vi "Write Scanner UDP Handle.vi"(8 "error in (no error)":errorcluster, 10 "HTTP response":string, 11 "PF_API in":refnum<class "PF_API.lvclass">) -> (0 "error out":errorcluster, 3 "PF_API out":refnum<class "PF_API.lvclass">)   [LabVIEW 2019, in "PF_API.lvclass"]
uses:
  PF_API.lvclass
  PF_API.lvclass/PF_API.ctl
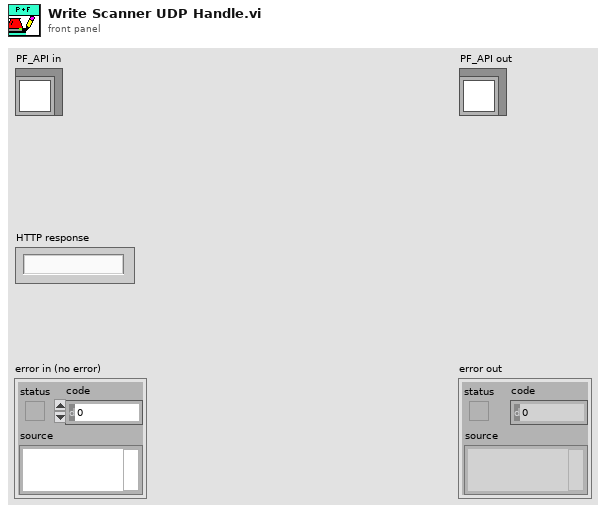
[diagram p1: front panel]
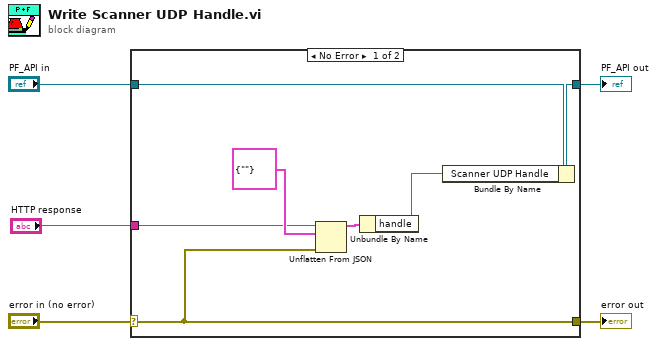
[diagram p0: block diagram]
diagram:
  n1 = case shown="No Error" "error in (no error)" {
    selector: "error in (no error)" -> [w8 w13]
    tunnel: [w8 w13] -> w4
    tunnel: [w11 w14] -> w2
    tunnel: "PF_API in" -> [w12 w14]
    tunnel: "HTTP response" -> [w9 _]
    frame No Error {
      n2 = Unflatten From JSON(JSON string=w9, type and defaults=cluster{"handle":string} {"handle"=""}, error in (no error)=w8) -> (value=w7:cluster{"handle":string})  [unwired: 4 in, 1 out]
      n3 = Unbundle By Name(w7) -> ("handle"=w6:string)
      n4 = Bundle By Name(cluster=w12, "Scanner UDP Handle"=w6) -> (w11:refnum<class "PF_API.lvclass">)
    }
    frame Error {
    }
  }
  "error out" <- w4
  "PF_API out" <- w2
